vi "Parse Header.vi"(8 "error in (no error)":errorcluster, 11 "Request in":refnum<class "Request.lvclass">) -> (0 "error out":errorcluster, 3 "Request out":refnum<class "Request.lvclass">)   [LabVIEW 2023, in "Request.lvclass"]
uses:
  Request.lvclass
  Request.lvclass/Request.ctl
  <vilib>/Utility/error.llb/Trim Whitespace One-Sided.vi
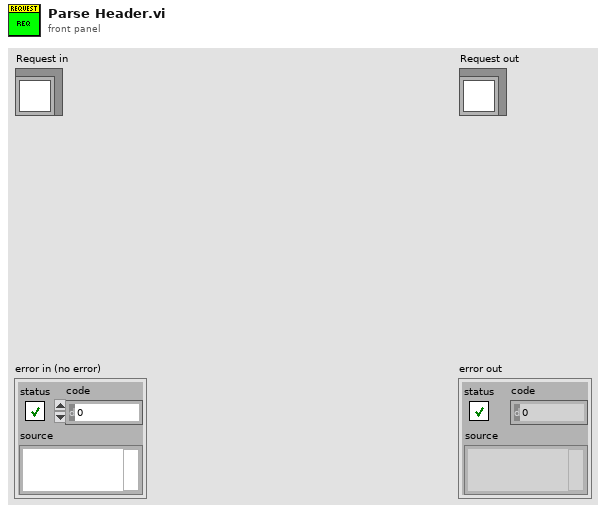
[diagram p1: front panel]
types:
  T1 = typedef "Request.ctl" = cluster{"Method":string, "URI":string, "Protocol":string, "Raw Path":string, "Query":string, "Fragment":string, "Raw Body":string, "Headers":variant, "Parameters":variant, "Body":variant, "Raw Header":string, "Path":string[]}
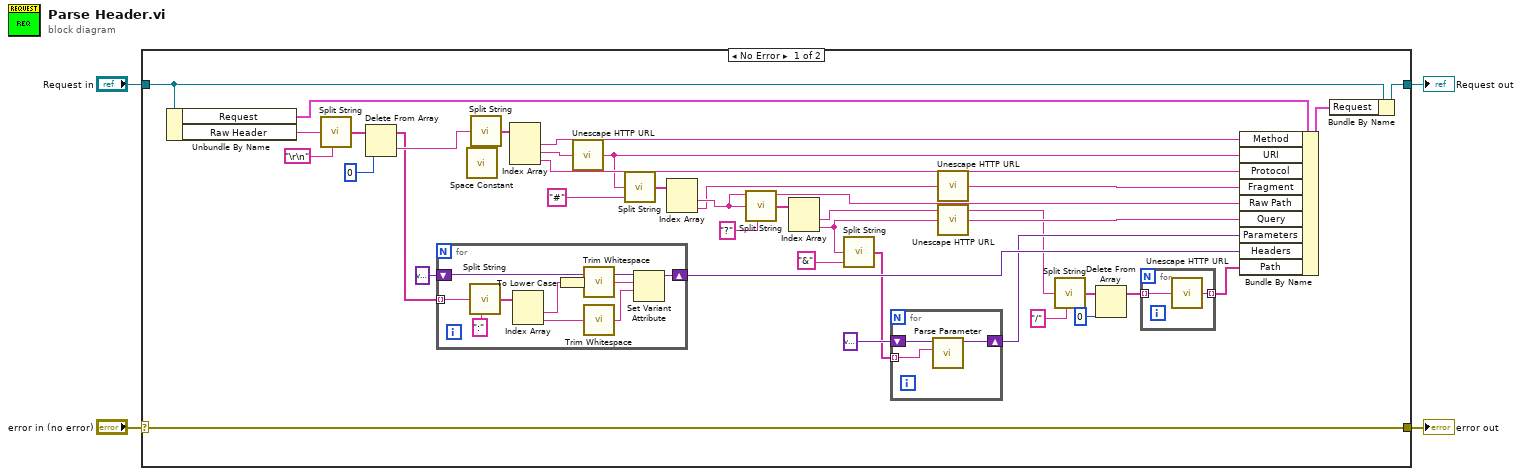
[diagram p0: block diagram]
diagram:
  n1 = case shown="No Error" "error in (no error)" {
    selector: "error in (no error)" -> [w20 w59]
    tunnel: [w20 w59] -> w3
    tunnel: [w41 w58] -> w1
    tunnel: "Request in" -> [w42 w58]
    frame No Error {
      n2 = Unbundle By Name(w42) -> ("Request"=w18:T1, "Raw Header"=w21:string)
      n3 = call "Split String.vi"("String"=w21, "Delimiter"="\r\n") -> ("Elements"=w39:string[])  [unwired: 7 in]
      n4 = Delete From Array(array=w39, index=0) -> (deleted portion=w37:string, array with subset deleted=w32:string[])  [unwired: 1 in]
      n5 = for {
        tunnel: w32 -> [w57] mode=indexing
        shift-right: [w54] -> w30
        shift-left: variant ("Request.Headers") -> [w55]
        n6 = call "Split String.vi"("String"=w57, "Delimiter"=":") -> ("Elements"=w53:string[])  [unwired: 7 in]
        n7 = Index Array(array=w53) -> (element #1=w52:string, element #2=w51:string)  [unwired: 2 in]
        n8 = To Lower Case(string=w52) -> (all lower case string=w48:string)
        n9 = call <vilib>:"Trim Whitespace.vi"("string"=w48) -> ("trimmed string"=w49:string)  [unwired: 1 in]
        n10 = call <vilib>:"Trim Whitespace.vi"("string"=w51) -> ("trimmed string"=w50:string)  [unwired: 1 in]
        n11 = Set Variant Attribute(Variant=w55, name=w49, value=w50) -> (Variant out=w54:variant)  [unwired: 1 in, 2 out]
      }
      n12 = call <vilib>:"Space Constant.vi"() -> ("String"=w36:string)
      n13 = call "Split String.vi"("String"=w37, "Delimiter"=w36) -> ("Elements"=w35:string[])  [unwired: 7 in]
      n14 = Index Array(array=w35) -> (element #1=w34:string, element #2=w6:string, element #3=w33:string)  [unwired: 3 in]
      n15 = call "Unescape HTTP URL.vi"("escaped string in"=w6) -> ("unescaped string out"=w5:string)
      n16 = call "Split String.vi"("String"=w5, "Delimiter"="#") -> ("Elements"=w28:string[])  [unwired: 7 in]
      n17 = Index Array(array=w28) -> (element #1=w17:string, element #2=w12:string)  [unwired: 2 in]
      n18 = call "Split String.vi"("String"=w17, "Delimiter"="?") -> ("Elements"=w26:string[])  [unwired: 7 in]
      n19 = Index Array(array=w26) -> (element #1=w7:string, element #2=w14:string)  [unwired: 2 in]
      n20 = call "Split String.vi"("String"=w14, "Delimiter"="&") -> ("Elements"=w23:string[])  [unwired: 7 in]
      n21 = for {
        tunnel: w23 -> [w45] mode=indexing
        shift-right: [w46] -> w22
        shift-left: variant ("Request.Headers") -> [w47]
        n22 = call "Parse Parameter.vi"("Parameter"=w45, "Request.Headers in"=w47) -> ("Request.Headers out"=w46:variant)  [unwired: 9 in]
      }
      n23 = call "Unescape HTTP URL.vi"("escaped string in"=w12) -> ("unescaped string out"=w11:string)
      n24 = call "Unescape HTTP URL.vi"("escaped string in"=w14) -> ("unescaped string out"=w13:string)
      n25 = call "Split String.vi"("String"=w7, "Delimiter"="/") -> ("Elements"=w10:string[])  [unwired: 7 in]
      n26 = Delete From Array(array=w10, index=0) -> (array with subset deleted=w9:string[])  [unwired: 1 in, 1 out]
      n27 = for {
        tunnel: w9 -> [w44] mode=indexing
        tunnel: [w43] -> w16 mode=indexing
        n28 = call "Unescape HTTP URL.vi"("escaped string in"=w44) -> ("unescaped string out"=w43:string)
      }
      n29 = Bundle By Name(cluster=w18, "Method"=w34, "URI"=w5, "Protocol"=w33, "Fragment"=w11, "Raw Path"=w17, "Query"=w13, "Parameters"=w22, "Headers"=w30, "Path"=w16) -> (w19:T1)
      n30 = Bundle By Name(cluster=w42, "Request"=w19) -> (w41:refnum<class "Request.lvclass">)
    }
    frame Error {
    }
  }
  "error out" <- w3
  "Request out" <- w1
